vi "TDMS Global.vi"() -> ()   [LabVIEW 2023]
panel:
  in  "FPGA":string="FPGA"
  in  "Left Offset":string="Left Offset"
  in  "Total Width":string="Total Width"
  in  "Bytes Per Image":string="Bytes Per Image"
  in  "Pixels Per Image":string="Pixels Per Image"
  in  "Reserve Size":string="Reserve Size"
  in  "Disable Buffering":string="Disable Buffering"
  in  "Async":string="Async"
  in  "Height":string="Height"
  in  "Width":string="Width"
  in  "Image Type":string="Image Type"
  in  "Channel Name":string="Image Data"
  in  "Group Name":string="Camera Acquisition"
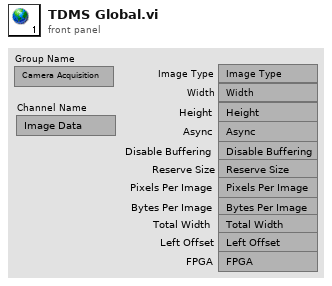
[diagram p1: front panel]
diagram:
